vi "ConfigureAdaptorr04.vi"() -> ()   [LabVIEW 2011]
doc: "The Basic Serial Read and Write example performs a Serial Port Read, a Serial Port Write, or a combination of these actions. The user selects the actions (read or write) on the front panel. If both are selected, the VI will write the data first, read data, and then close the VISA session that is opened to the port. This VI will wait until the specified number of bytes is received at the port or until a termination character is read.\n\nINSTRUCTIONS:\n1) Select the serial resource and configuration parameters (baud rate, data bits, parity, stop bits, flow control).\n2) Select the operations to be performed. \n3) Connect the serial port to your device. If no device is available, perform a loopback test by doing one of the following. Short pins 2 and 3 on a RS-232 cable or short pin 4 to pin 8 and pin 5 to pin 9 on a RS-485/422 cable. \n4) Run the VI to see the data read. (The \"read string\" will match the \"string to write\" if a loopback test was performed.)\n\nNote: The parameters set for the serial port must match the parameters of the connected instrument or device. In this example, the bytes to read parameter specifies the number of bytes that the serial port reads. If there were more bytes at the port than the number specified in bytes to read, those bytes would not be read. Also, if you specify to read more bytes than the number of bytes actually read, you might receive a timeout error message.\n\nOn the block diagram, the Configure Serial Port VI sets the configuration parameters. The front panel displays the controls used to configure the basic parameters, such as baud rate, data bits, and parity. Constants configure the other parameters the user probably does not need set. After the VISA Configure Serial Port VI opens the VISA session and configures the port, the VI passes the VISA resource name to other VIs that perform operations on that VISA resource. The VISA Write function sends a command to the serial device and the VISA Read function returns data based on the command. The VISA Close function then closes the reference to the serial device. It is important to close the reference; otherwise communication through with that port through protocols other than VISA might not be possible."
panel:
  out "concatenated string":string
  in  "Trip Point 1(Torr)":dbl=700.0
  in  "Tab Control":enum32{"I/O", "AdapTorr"}(tab)
  in  "delay before read (ms)":u32=500
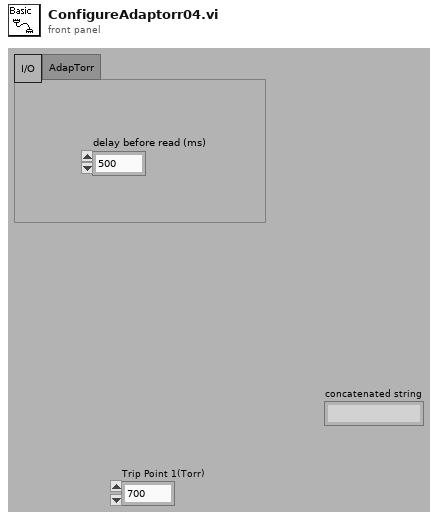
[diagram p1: front panel]
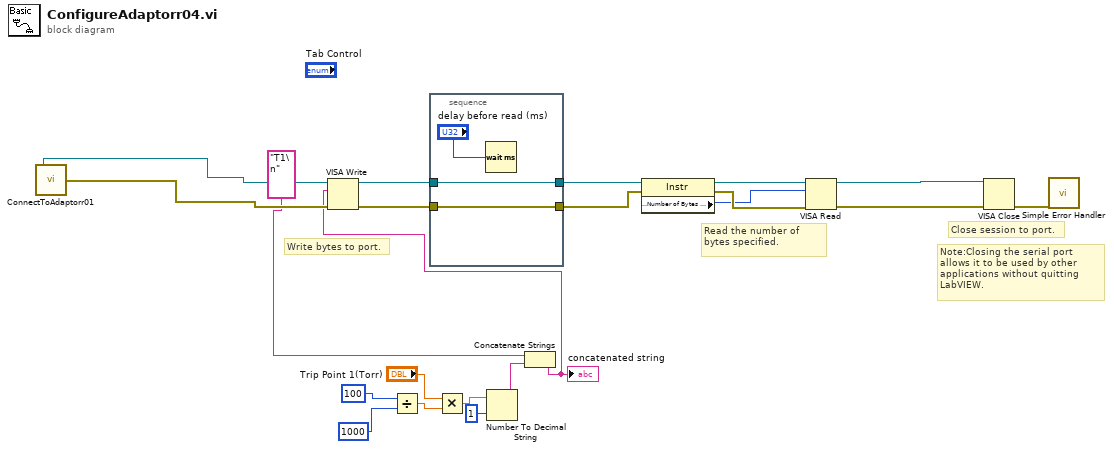
[diagram p0: block diagram]
diagram:
  # "Write bytes to port."
  # "Read the number of bytes specified."
  # "Note:Closing the serial port allows it to be used by other applications without quitting LabVIEW."
  # "Close session to port."
  n1 = call "ConnectToAdaptorr01.vi"() -> ("error out"=w10:errorcluster, "VISA resource name out"=w11:refnum<visa-resource-name>)  [unwired: 1 in]
  n2 = Divide(x=100, y=1000) -> (x/y=w7:dbl)
  n3 = Multiply(x="Trip Point 1(Torr)", y=w7) -> (x*y=w5:dbl)
  n4 = Number To Decimal String(number=w5, width (-)=i16 1) -> (decimal integer string=w3:string)
  n5 = Concatenate Strings("T1\n" ("string to write"), w3) -> (w2:string)
  "concatenated string" <- w2
  n6 = VISA Write(VISA resource name=w11, write buffer=w2, error in (no error)=w10) -> (VISA resource name out=w16:refnum<visa-resource-name>, error out=w18:errorcluster)  [unwired: 1 out]
  n7 = stacked-sequence {
    tunnel: w18 -> [w24]
    tunnel: [w24] -> w17
    tunnel: w16 -> [w23]
    tunnel: [w23] -> w15
    frame #0 {
      n8 = Wait (ms)(milliseconds to wait="delay before read (ms)") -> ()  [unwired: 1 out]
    }
  }
  n9 = property class="Instr"(reference=w15, error in=w17) -> (reference out=w14:refnum<visa-resource-name>, error out=w13:errorcluster, "Serial Settings:Number of Bytes at Serial Port"=w12:u32)
  n10 = VISA Read(VISA resource name=w14, byte count=w12, error in (no error)=w13) -> (VISA resource name out=w20:refnum<visa-resource-name>, error out=w21:errorcluster)  [unwired: 2 out]
  n11 = VISA Close(VISA resource name=w20, error in (no error)=w21) -> (error out=w19:errorcluster)
  n12 = call <vilib>:"Simple Error Handler.vi"("error in (no error)"=w19) -> ()  [unwired: 1 in, 8 out]
